vi "RunProcMsg.vi"(0 "reference in":refnum<class "Proccess.lvclass">, 5 "error in (no error)":errorcluster) -> (14 "reference out":refnum<class "Proccess.lvclass">, 19 "error out":errorcluster)   [LabVIEW 2019, in "Proccess.lvclass"]
uses:
  Proccess.lvclass
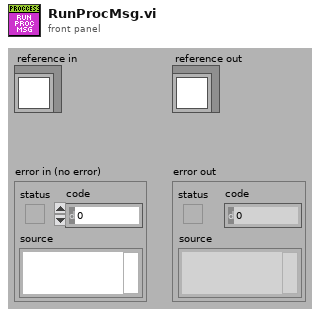
[diagram p1: front panel]
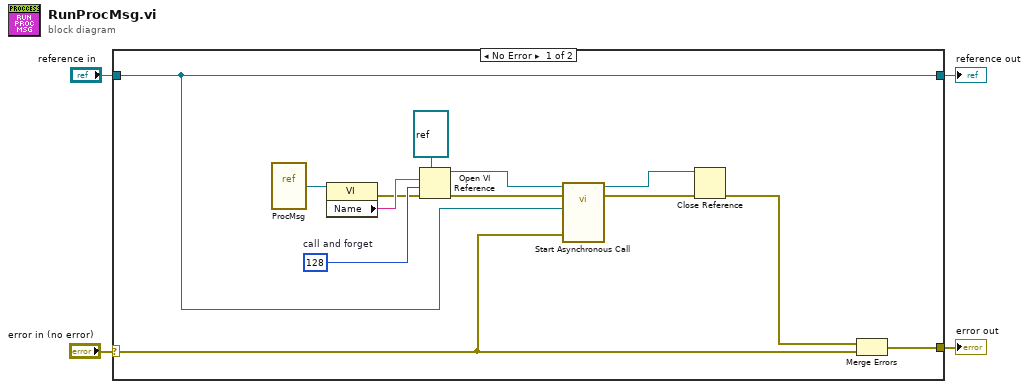
[diagram p0: block diagram]
diagram:
  n1 = case shown="No Error" "error in (no error)" {
    selector: "error in (no error)" -> [w9 w19]
    tunnel: [w7 w19] -> w3
    tunnel: [w8 w18] -> w1
    tunnel: "reference in" -> [w8 w18]
    frame No Error {
      w17 = 128  # call and forget
      n2 = vi-ref "ProcMsg.vi"() -> (w12:refnum<vi>)
      n3 = property class="VI"(reference=w12) -> (error out=w10:errorcluster, "Name"=w11:string)  [unwired: 1 in, 1 out]
      n4 = Open VI Reference(type specifier VI Refnum (for type only)=refnum<vi> refnum, vi path=w11, options=w17, error in (no error)=w10) -> (vi reference=w5:refnum<vi>, error out=w15:errorcluster)  [unwired: 2 in]
      n5 = call-by-ref "Start Asynchronous Call"(reference=w5, error in=w15, "reference in"=w8, 5:"error in (no error)"=w9) -> (reference out=w13:refnum<vi>, error out=w14:errorcluster)  [unwired: 16 in, 2 out]
      n6 = Close Reference(reference=w13, error in (no error)=w14) -> (error out=w6:errorcluster)
      n7 = Merge Errors(w6, w9) -> (w7:errorcluster)
    }
    frame Error {
    }
  }
  "error out" <- w3
  "reference out" <- w1
